vi "SetParam.vi"(8 "error in (no error)":errorcluster caption="entrée d'erreur (pas d'erreur)", 10 "mean_gamma_deviance":cluster{"sample_weight":dbl[]}, 11 "Mean_Gamma_Deviance.lvclass":refnum<class "Mean_Gamma_Deviance.lvclass">) -> (0 "error out":errorcluster caption="sortie d'erreur", 3 "Mean_Gamma_Deviance.lvclass":refnum<class "Mean_Gamma_Deviance.lvclass">)   [LabVIEW 2020, in "Mean_Gamma_Deviance.lvclass"]
doc: "Set Parameters"
uses:
  Mean_Gamma_Deviance.lvclass
  Mean_Gamma_Deviance.lvclass/Mean_Gamma_Deviance.ctl
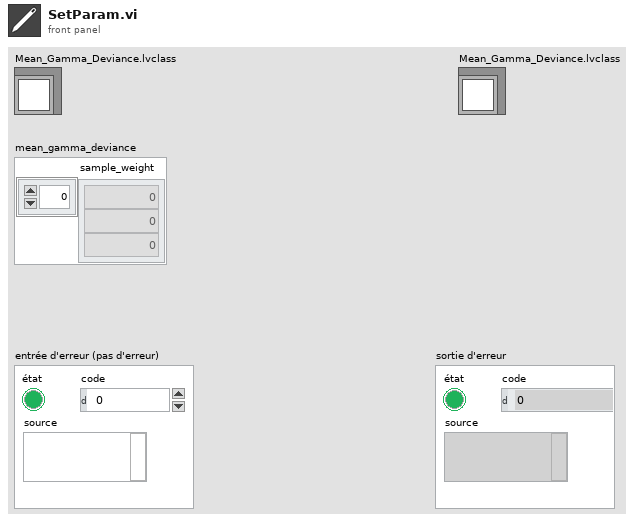
[diagram p1: front panel]
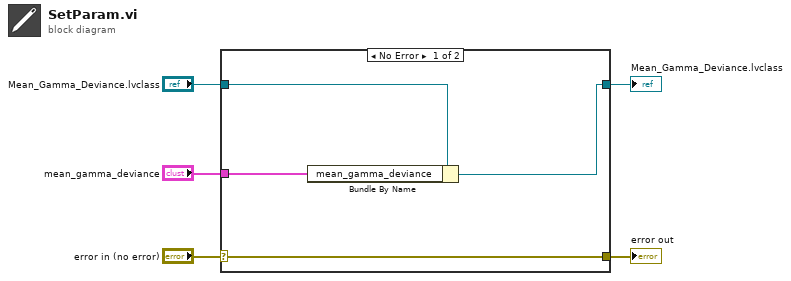
[diagram p0: block diagram]
diagram:
  n1 = case shown="No Error" "error in (no error)" {
    selector: "error in (no error)" -> [w9 w10]
    tunnel: [w9 w10] -> w4
    tunnel: [w7 w11] -> w2
    tunnel: "Mean_Gamma_Deviance.lvclass" -> [w8 w11]
    tunnel: "mean_gamma_deviance" -> [w6 _]
    frame No Error {
      n2 = Bundle By Name(cluster=w8, "mean_gamma_deviance"=w6) -> (w7:refnum<class "Mean_Gamma_Deviance.lvclass">)
    }
    frame Error {
    }
  }
  "error out" <- w4
  "Mean_Gamma_Deviance.lvclass" <- w2
